vi "Main_BX.vi"() -> ()   [LabVIEW 2017]
panel:
  in  "Tab Control":enum32{"BangXiang_SaveData"}(tab)
  out "Post test show":dbl[][](graph)
  in  "Manule Input 2":dbl(slide) scale=0.0..10.0
  in  "Manule Input 1":dbl(slide) scale=0.0..10.0
  out "File Name":string
  in  "# of Expermintens":string="99"
  in  "# of Version":string="99"
  in  "Test Theme":string="Bangxiang"
  out "Real time show":cluster{"Double":dbl, "Double":dbl}(graph)
  in  "Save and Stop":bool
  # "Usage: \n\n1. Run. \n2. Manuipulate two slide inputs\n3. Stop. And check the subfolder ...\\data\\[File Name]"
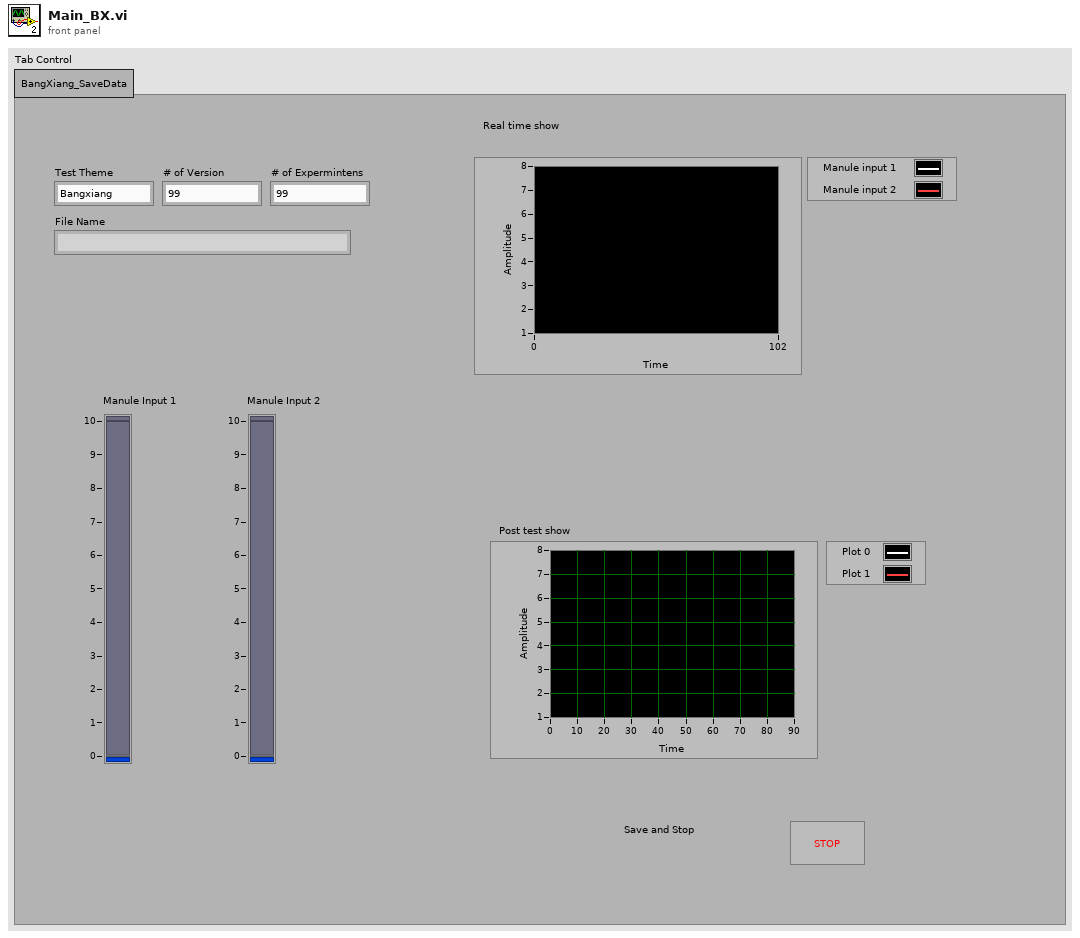
[diagram p1: front panel]
types:
  T1 = enum16{"open", "replace", "create", "open or create", "replace or create", "replace or create with confirmation"}
  T2 = cluster{"Manule Input 1":dbl, "Manule Input 2":dbl}
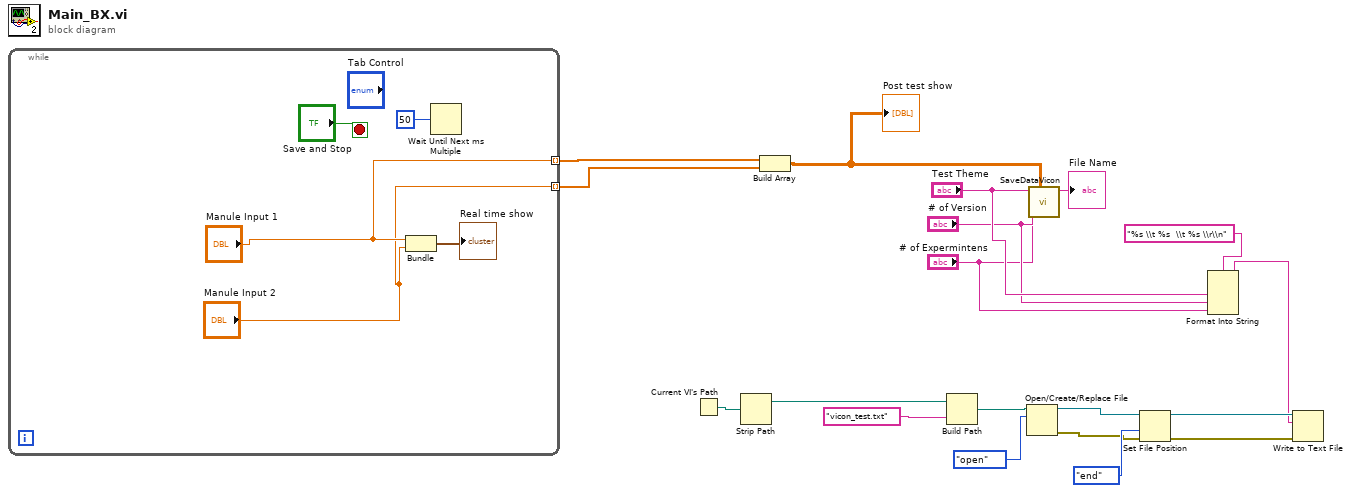
[diagram p0: block diagram]
diagram:
  n1 = while {
    tunnel: ["Manule Input 1"] -> w3 mode=indexing
    tunnel: ["Manule Input 2"] -> w4 mode=indexing
    stop <- "Save and Stop" stop-if-true
    n2 = Bundle("Manule Input 1"="Manule Input 1", "Manule Input 2"="Manule Input 2") -> (→"Real time show":T2)  [unwired: 1 in]
    n3 = Wait Until Next ms Multiple(millisecond multiple=u32 50) -> ()  [unwired: 1 out]
  }
  n4 = Current VI's Path() -> (path=w18:path)
  n5 = Strip Path(path=w18) -> (stripped path=w17:path)  [unwired: 1 out]
  n6 = Build Array(w3, w4) -> (w2:dbl[][])
  "Post test show" <- w2
  n7 = Build Path(base path=w17, name or relative path="vicon_test.txt") -> (appended path=w9:path)
  n8 = Open/Create/Replace File(file path (use dialog)=w9, operation (0:open)=T1."open") -> (refnum out=w13:refnum<file>, error out=w11:errorcluster)  [unwired: 4 in, 1 out]
  n9 = call "SaveDataVicon.vi"("Array"=w2, "# of Expermintens"="# of Expermintens", "# of Version"="# of Version", "Test Theme"="Test Theme") -> ("File Name"=→"File Name":string)  [unwired: 7 in]
  n10 = Set File Position(refnum=w13, from (0:start)=enum16{"start", "end", "current"}."end", error in=w11) -> (refnum out=w15:refnum<file>, error out=w10:errorcluster)  [unwired: 1 in]
  n11 = Format Into String(format string="%s \\t %s  \\t %s \\r\\n" ("prompt (Choose or enter file path)"), "Test Theme", "# of Version", "# of Expermintens") -> (resulting string=w7:string)  [unwired: 2 in, 1 out]
  n12 = Write to Text File(file (use dialog)=w15, text=w7, error in=w10) -> ()  [unwired: 1 in, 3 out]
